vi "writeHighlowArduino.vi"() -> ()   [LabVIEW 2018]
uses:
  <vilib>/LabVIEW Interface for Arduino/Type Defs/Pin Mode.ctl
  <vilib>/LabVIEW Interface for Arduino/LabVIEW Interface for Arduino.lvlib
panel:
  in  "stop":bool
  in  "Start step":u8(slide) scale=0.0..1.0
  in  "Direction":u8(slide) scale=0.0..1.0
  in  "VISA resource":refnum<visa-resource-name>
  out "error out":errorcluster
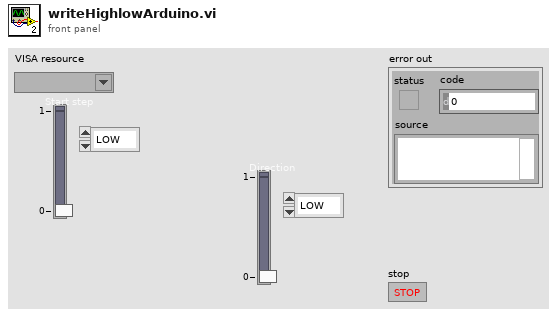
[diagram p1: front panel]
types:
  T1 = typedef "LabVIEW Interface for Arduino.lvlib/Arduino Resource.ctl" = cluster{"VISA resource":refnum<visa-resource-name>, "Board Type":T2, "Connection Type":enum8{"USB / Serial"}, "Bytes Per Packet (15)":u8}
  T2 = typedef "LabVIEW Interface for Arduino.lvlib/Board Type.ctl" = enum16{"Uno", "Dimuelanove w/Atmega 328", "Mega 2560"}
  T3 = typedef "LabVIEW Interface for Arduino.lvlib/Pin Mode.ctl" = enum8{"Input", "Output"}
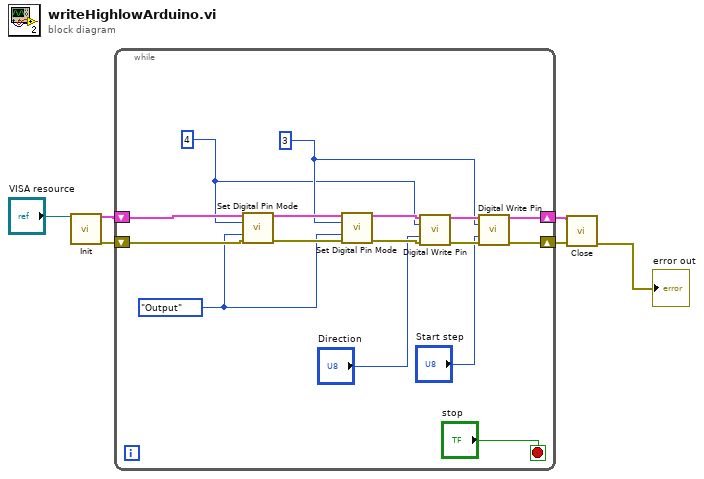
[diagram p0: block diagram]
diagram:
  n1 = call <vilib>:"Init.vi"("VISA resource"="VISA resource") -> ("Arduino Resource"=w6:T1, "error out"=w5:errorcluster)  [unwired: 17 in]
  n2 = while {
    shift-right: [w14] -> w4
    shift-left: w6 -> [w22]
    shift-right: [w13] -> w3
    shift-left: w5 -> [w20]
    stop <- "stop" stop-if-true
    w10 = Pin_Mode."Output" ("Pin Mode (Input)")
    w12 = u8 3 ("Digital I/O Pin")
    w11 = u8 4 ("Digital I/O Pin")
    n3 = call <vilib>:"Set Digital Pin Mode.vi"("Arduino Resource"=w22, "Digital I/O Pin"=w11, "Pin Mode (Input)"=w10, "error in"=w20) -> ("Arduino Resource"=w21:T1, "error out"=w19:errorcluster)  [unwired: 10 in]
    n4 = call <vilib>:"Set Digital Pin Mode.vi"("Arduino Resource"=w21, "Digital I/O Pin"=w12, "Pin Mode (Input)"=w10, "error in"=w19) -> ("Arduino Resource"=w18:T1, "error out"=w17:errorcluster)  [unwired: 10 in]
    n5 = call <vilib>:"Digital Write Pin.vi"("Arduino Resource"=w18, "Digital I/O Pin (0)"=w11, "Value (0)"="Direction", "error in"=w17) -> ("Arduino Resource"=w16:T1, "error out"=w15:errorcluster)  [unwired: 10 in]
    n6 = call <vilib>:"Digital Write Pin.vi"("Arduino Resource"=w16, "Digital I/O Pin (0)"=w12, "Value (0)"="Start step", "error in"=w15) -> ("Arduino Resource"=w14:T1, "error out"=w13:errorcluster)  [unwired: 10 in]
  }
  n7 = call <vilib>:"Close.vi"("Arduino Resource"=w4, "error in"=w3) -> ("error out"=→"error out":errorcluster)  [unwired: 13 in]
